vi "Mouse Down.vi"(8 "error in":errorcluster, 10 "Double Click":bool, 11 "Data in":T1={"Class"={"Ants"=refnum, "Layer"=refnum, "Templates"=refnum, "Icon"=refnum, "Glyph"=refnum, "Settings"=refnum, "Tools"=refnum}, "Ref"={"Add Layer"=refnum, "Remove Layer"=refnum, "Line Text"=[], "Body Text Spec"=refnum, "DNL_Font"=refnum, "glyph path str"=refnum, "templates path str"=refnum, "Arrow Up"=refnum, "Arrow Down"=refnum, "IE VI Ref"=refnum, "Glyphs tree"=refnum, "Templates tree"=refnum, "Layer Icon Text"=refnum, "Layer Template"=refnum, "Clipboard"=refnum, "BW icon in"=refnum, "Color icon in"=refnum, "Layer Clust"=refnum, "Body Text"=refnum, "DNL_Framework Templates"=refnum, "Search Templates"=refnum, "TextMarker"=refnum, "Tab Control"=refnum, "Search Glyphs"=refnum, "Line Color"=refnum, "DNL_Glyphs []"=refnum, "Fill Color"=refnum, "Tools"=refnum, "Glyphs tree"=refnum, "Icon"=refnum, "Preview"=refnum, "Ants"=refnum, "Terminals"=refnum, "menu reference"=refnum, "LayerNames"=[], "GlyphLoadAnimation"=refnum, "TemplateLoadAnimation"=refnum, "refreshGlyphs"=refnum, "refreshTemplates"=refnum}, "Support"={"AntsRect"={"left"=0, "top"=0, "right"=0, "bottom"=0}, "Mouse Move Coords"={"Horizontal"=0, "Vertical"=0}, "Mouse Down Coords"={"Horizontal"=0, "Vertical"=0}, "Temp Coord"={"Horizontal"=0, "Vertical"=0}, "Action"=enum."Default", "Edge Color"=4914962, "Fill Color"=16860, "Mouse Down?"=FALSE, "Draft Mode?"=FALSE, "Temp Icon"=bytes[3102], "CTRL Pressed"=FALSE, "Move Selection?"=FALSE, "AntsRect Orig"={"left"=0, "top"=0, "right"=0, "bottom"=0}, "Text"="", "TM Set?"=FALSE, "Mouse inside icon?"=FALSE, "Tool (old value)"=0, "Pencil Move Color"=0, "Swap Colors?"=FALSE, "Shift pressed?"=FALSE}}) -> (0 "error out":errorcluster, 3 "Data out":T1={"Class"={"Ants"=refnum, "Layer"=refnum, "Templates"=refnum, "Icon"=refnum, "Glyph"=refnum, "Settings"=refnum, "Tools"=refnum}, "Ref"={"Add Layer"=refnum, "Remove Layer"=refnum, "Line Text"=[], "Body Text Spec"=refnum, "DNL_Font"=refnum, "glyph path str"=refnum, "templates path str"=refnum, "Arrow Up"=refnum, "Arrow Down"=refnum, "IE VI Ref"=refnum, "Glyphs tree"=refnum, "Templates tree"=refnum, "Layer Icon Text"=refnum, "Layer Template"=refnum, "Clipboard"=refnum, "BW icon in"=refnum, "Color icon in"=refnum, "Layer Clust"=refnum, "Body Text"=refnum, "DNL_Framework Templates"=refnum, "Search Templates"=refnum, "TextMarker"=refnum, "Tab Control"=refnum, "Search Glyphs"=refnum, "Line Color"=refnum, "DNL_Glyphs []"=refnum, "Fill Color"=refnum, "Tools"=refnum, "Glyphs tree"=refnum, "Icon"=refnum, "Preview"=refnum, "Ants"=refnum, "Terminals"=refnum, "menu reference"=refnum, "LayerNames"=[], "GlyphLoadAnimation"=refnum, "TemplateLoadAnimation"=refnum, "refreshGlyphs"=refnum, "refreshTemplates"=refnum}, "Support"={"AntsRect"={"left"=0, "top"=0, "right"=0, "bottom"=0}, "Mouse Move Coords"={"Horizontal"=0, "Vertical"=0}, "Mouse Down Coords"={"Horizontal"=0, "Vertical"=0}, "Temp Coord"={"Horizontal"=0, "Vertical"=0}, "Action"=enum."Default", "Edge Color"=4914962, "Fill Color"=16860, "Mouse Down?"=FALSE, "Draft Mode?"=FALSE, "Temp Icon"=bytes[3102], "CTRL Pressed"=FALSE, "Move Selection?"=FALSE, "AntsRect Orig"={"left"=0, "top"=0, "right"=0, "bottom"=0}, "Text"="", "TM Set?"=FALSE, "Mouse inside icon?"=FALSE, "Tool (old value)"=0, "Pencil Move Color"=0, "Swap Colors?"=FALSE, "Shift pressed?"=FALSE}})   [LabVIEW 2021]
uses:
  <resource>/plugins/NIIconEditor/Controls/IE Data.ctl
  <resource>/plugins/NIIconEditor/Class/Ants/Ants.lvclass
  <resource>/plugins/NIIconEditor/Class/FakedArray/FakedArray.lvclass
  <resource>/plugins/NIIconEditor/Class/Icon Library/Glyph.lvclass
  <resource>/plugins/NIIconEditor/Class/Settings/Settings.lvclass
  <resource>/plugins/NIIconEditor/Class/Tools/Tools Paint.lvclass
  <vilib>/LabVIEW Icon API/lv_icon/Classes/Icon/Icon.lvclass
  <resource>/plugins/NIIconEditor/Controls/IE Classes.ctl
  <resource>/plugins/NIIconEditor/Controls/References Cluster.ctl
  <resource>/plugins/NIIconEditor/Controls/SupportClass.ctl
  <vilib>/Utility/miscctls.llb/LVPoint32TypeDef.ctl
  <resource>/plugins/NIIconEditor/Controls/SupportClass_Action.ctl
  <vilib>/LabVIEW Icon API/lv_icon/Controls/IEColor.ctl
  <vilib>/LabVIEW Icon API/lv_icon/Controls/LayerType.ctl
  <vilib>/LabVIEW Icon API/lv_icon/Classes/Layer/Layer.lvclass
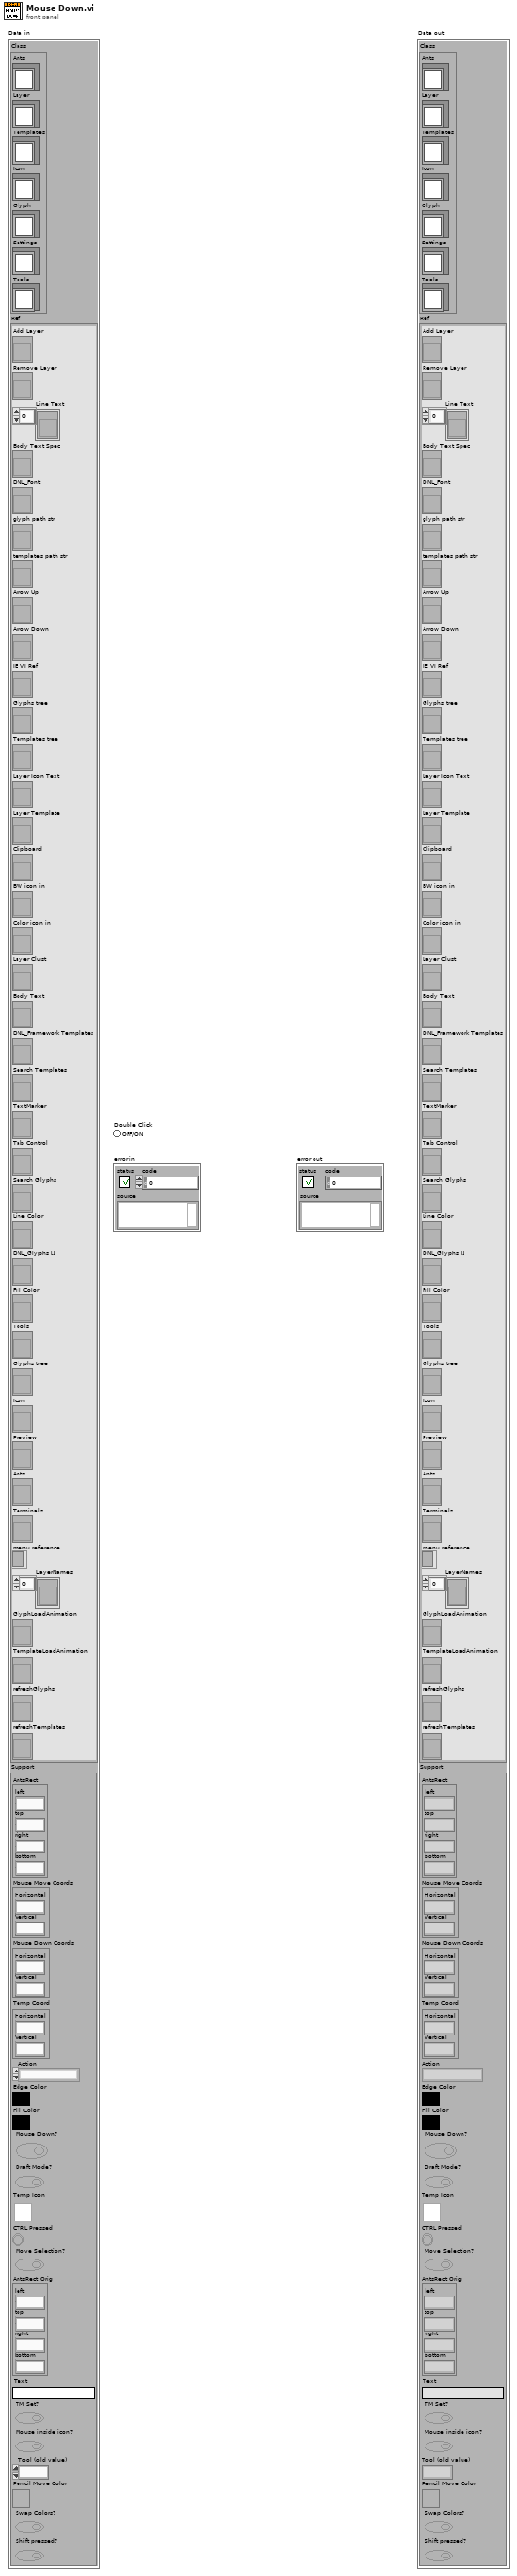
[diagram p1: front panel]
types:
  T1 = typedef "IE Data.ctl" = cluster{"Class":T2, "Ref":T3, "Support":T4}
  T2 = typedef "IE Classes.ctl" = cluster{"Ants":refnum<class "Ants.lvclass">, "Layer":refnum<class "FakedArray.lvclass">, "Templates":refnum<class "FakedArray.lvclass">, "Icon":refnum<class "Icon.lvclass">, "Glyph":refnum<class "Glyph.lvclass">, "Settings":refnum<class "Settings.lvclass">, "Tools":refnum<class "Tools Paint.lvclass">}
  T3 = typedef "References Cluster.ctl" = cluster{"Add Layer":refnum<vi>, "Remove Layer":refnum<vi>, "Line Text":refnum<vi>[], "Body Text Spec":refnum<vi>, "DNL_Font":refnum<vi>, "glyph path str":refnum<vi>, "templates path str":refnum<vi>, "Arrow Up":refnum<vi>, "Arrow Down":refnum<vi>, "IE VI Ref":refnum<vi>, "Glyphs tree":refnum<vi>, "Templates tree":refnum<vi>, "Layer Icon Text":refnum<vi>, "Layer Template":refnum<vi>, "Clipboard":refnum<vi>, "BW icon in":refnum<vi>, "Color icon in":refnum<vi>, "Layer Clust":refnum<vi>, "Body Text":refnum<vi>, "DNL_Framework Templates":refnum<vi>, "Search Templates":refnum<vi>, "TextMarker":refnum<vi>, "Tab Control":refnum<vi>, "Search Glyphs":refnum<vi>, "Line Color":refnum<vi>, "DNL_Glyphs []":refnum<vi>, "Fill Color":refnum<vi>, "Tools":refnum<vi>, "Glyphs tree":refnum<vi>, "Icon":refnum<vi>, "Preview":refnum<vi>, "Ants":refnum<vi>, "Terminals":refnum<vi>, "menu reference":refnum<k9>, "LayerNames":refnum<vi>[], "GlyphLoadAnimation":refnum<vi>, "TemplateLoadAnimation":refnum<vi>, "refreshGlyphs":refnum<vi>, "refreshTemplates":refnum<vi>}
  T4 = typedef "SupportClass.ctl" = cluster{"AntsRect":cluster{"left":i16, "top":i16, "right":i16, "bottom":i16}, "Mouse Move Coords":T5, "Mouse Down Coords":T5, "Temp Coord":T5, "Action":T6, "Edge Color":T7, "Fill Color":T7, "Mouse Down?":bool, "Draft Mode?":bool, "Temp Icon":picture, "CTRL Pressed":bool, "Move Selection?":bool, "AntsRect Orig":cluster{"left":i16, "top":i16, "right":i16, "bottom":i16}, "Text":string, "TM Set?":bool, "Mouse inside icon?":bool, "Tool (old value)":u32, "Pencil Move Color":u32, "Swap Colors?":bool, "Shift pressed?":bool}
  T5 = typedef "LVPoint32TypeDef.ctl" = cluster{"Horizontal":i32, "Vertical":i32}
  T6 = typedef "SupportClass_Action.ctl" = enum16{"Default", "Move Selection", "Glyph Library", "Tool"}
  T7 = typedef "IEColor.ctl" = u32
  T8 = typedef "LayerType.ctl" = enum16{"Graphic", "Text", "Tool", "Graphic Drop"}
  T9 = cluster{"left":i16, "top":i16, "right":i16, "bottom":i16}
  T10 = typedef "Tools.ctl" = enum32{"Pencil", "Line", "Dropper", "Fill", "Rectangle", "Filled Rectangle", "Ellipse", "Filled Ellipse", "Eraser", "Text", "Select", "Move"}
  T11 = typedef "INI.ctl" = cluster{"Show Layer Tab?":bool, "Show Terminals?":bool, "Text":cluster{"Font":T12, "Alignment":T13, "Size":T14}, "3rd party Templates":cluster{"Store 3rd party Templates?":bool, "Folder Name":string}, "Merge user layers on commit":bool, "Body Text":T15, "Fill Color":T7, "Edge Color":T7, "Tab":u16, "Tool":T10, "Disable Layers?":bool}
  T12 = typedef "Font.ctl" = string
  T13 = typedef "Alignment.ctl" = u16
  T14 = typedef "Font Size.ctl" = u8
  T15 = typedef "BodyText.ctl" = cluster{"Line 1 text":string, "Line 2 text":string, "Line 3 text":string, "Line 4 text":string, "Line 1 color":u32, "Line 2 color":u32, "Line 3 color":u32, "Line 4 color":u32, "Body Text Spec":cluster{"Font":T12, "Alignment":T13, "Size":u8}, "Center text vertically":bool, "Capitalize Text":bool}
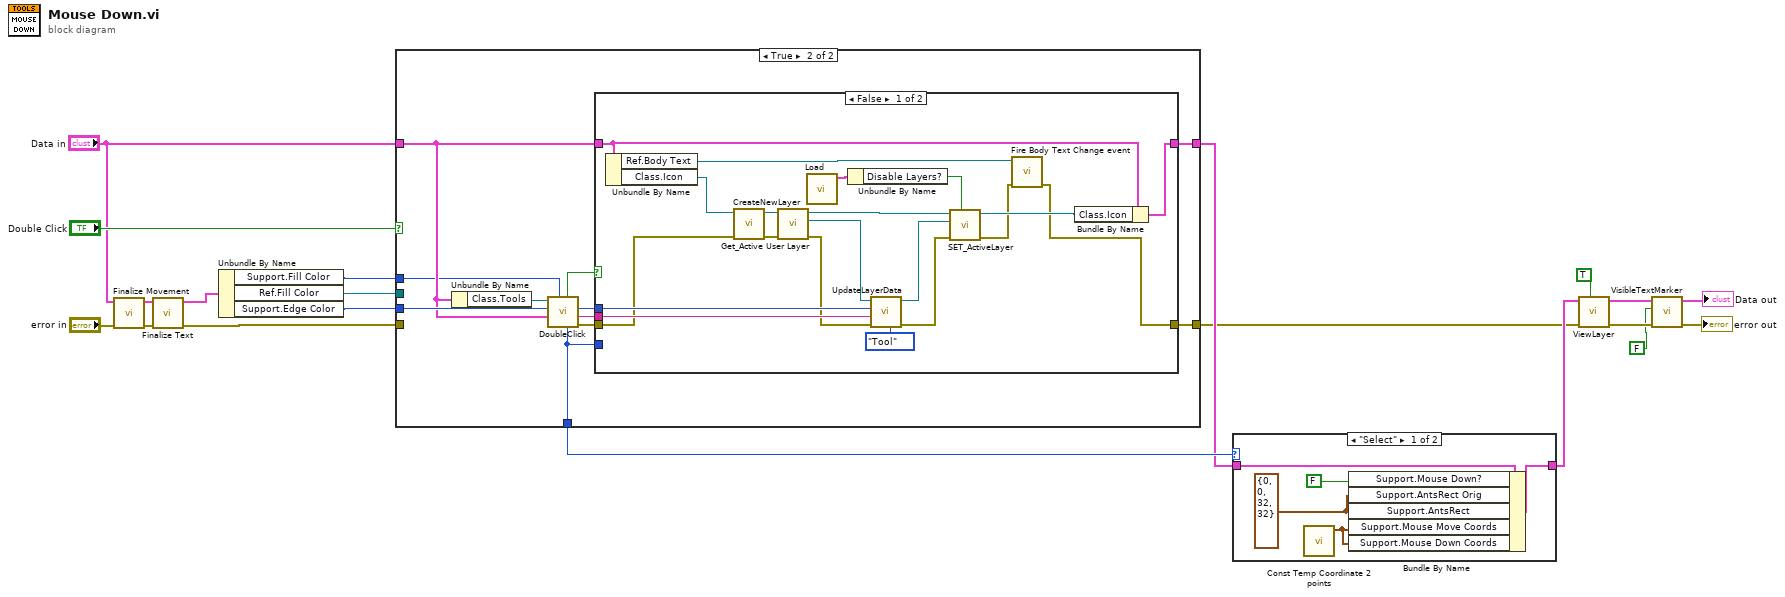
[diagram p0: block diagram]
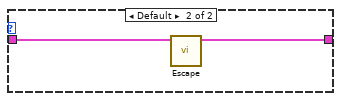
[diagram p2: hidden frame]
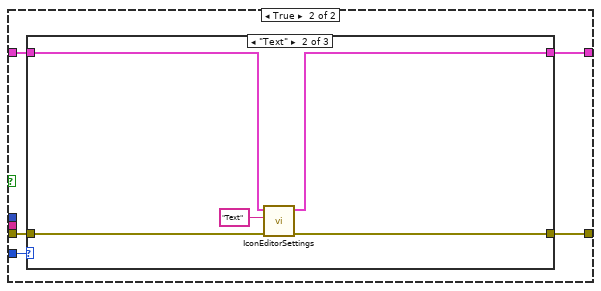
[diagram p4: hidden frame]
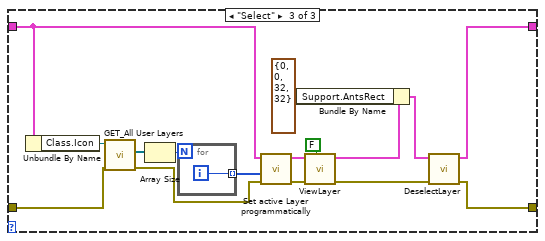
[diagram p6: hidden frame]
diagram:
  n1 = call <resource>:"Finalize Movement.vi"("error in (no error)"="error in", "Data in"="Data in") -> ("error out"=w13:errorcluster, "Data out"=w11:T1)  [unwired: 1 in, 7 out]
  n2 = call <resource>:"Finalize Text.vi"("error in (no error)"=w13, "Data in"=w11) -> ("error out"=w9:errorcluster, "Data out"=w10:T1)  [unwired: 8 out]
  n3 = Unbundle By Name(w10) -> ("Support.Fill Color"=w1:T7, "Ref.Fill Color"=w17:refnum<vi>, "Support.Edge Color"=w19:T7)
  n4 = case shown="True" "Double Click" {
    tunnel: w9 -> [w22 _]
    tunnel: w19 -> [_ w33]
    tunnel: [w22 w31] -> w2
    tunnel: [_ w27] -> w20
    tunnel: w17 -> [_ _]
    tunnel: "Data in" -> [w21 w25]
    tunnel: [w21 w24] -> w3
    tunnel: w1 -> [_ w23]
    frame False {
    }
    frame True {
      n5 = Unbundle By Name(w25) -> ("Class.Tools"=w26:refnum<class "Tools Paint.lvclass">)
      n6 = call <resource>:"DoubleClick.vi"("Fill Color"=w23, "Data in"=w25, "Edge Color"=w33, "Tools Paint in"=w26) -> ("error out"=w32:errorcluster, "Name"=w29:string, "new picture"=w30:picture, "Active Tool"=w27:T10, "Invalid Picture?"=w28:bool)  [unwired: 1 in, 2 out]
      n7 = case shown="False" w28 {
        tunnel: w32 -> [w50 w57]
        tunnel: [w37 w56] -> w31
        tunnel: w30 -> [w53 _]
        tunnel: w29 -> [w52 _]
        tunnel: w27 -> [_ w58]
        tunnel: w25 -> [w39 w55]
        tunnel: [w51 w54] -> w24
        frame False {
          n8 = Unbundle By Name(w39) -> ("Ref.Body Text"=w36:refnum<vi>, "Class.Icon"=w41:refnum<class "Icon.lvclass">)
          n9 = call <vilib>:"CreateNewLayer.vi"("error in"=w50, "Icon.lvclass"=w41) -> ("error out"=w49:errorcluster, "Icon.lvclass out"=w48:refnum<class "Icon.lvclass">)  [unwired: 3 in, 5 out]
          n10 = call-dynamic "Get_Active User Layer.vi"("error in (no error)"=w49, "Icon in"=w48) -> ("error out"=w46:errorcluster, "Layer.lvclass"=w45:refnum<class "Layer.lvclass">, "Icon out"=w47:refnum<class "Icon.lvclass">)  [unwired: 7 out]
          n11 = call <resource>:"Load.vi"() -> ("INI Data"=w35:T11)  [unwired: 2 in, 9 out]
          n12 = Unbundle By Name(w35) -> ("Disable Layers?"=w34:bool)
          n13 = call <vilib>:"UpdateLayerData.vi"("Type"=LayerType."Tool", "error in"=w46, "LayerName"=w52, "new picture"=w53, "Active Layer"=w45) -> ("error out"=w43:errorcluster, "Layer.lvclass out"=w44:refnum<class "Layer.lvclass">)  [unwired: 3 in, 2 out]
          n14 = call-dynamic "SET_ActiveLayer.vi"("Combine User Layers?"=w34, "error in (no error)"=w43, "Layer.lvclass"=w44, "Icon.lvclass in"=w47) -> ("error out"=w38:errorcluster, "Icon.lvclass out"=w40:refnum<class "Icon.lvclass">)  [unwired: 6 out]
          n15 = call <resource>:"Fire Body Text Change event.vi"("error in"=w38, "Ref.Body Text"=w36) -> ("error out"=w37:errorcluster)  [unwired: 2 in, 7 out]
          n16 = Bundle By Name(cluster=w39, "Class.Icon"=w40) -> (w51:T1)
        }
        frame True {
          n17 = case shown="\"Text\"" w58 {
            tunnel: w57 -> [w60 w65 w73]
            tunnel: [w60 w62 w66] -> w56
            tunnel: w55 -> [w59 w63 w72]
            tunnel: [w59 w61 w67] -> w54
            frame "Ellipse", Default {
            }
            frame "Text" {
              n18 = call <resource>:"IconEditorSettings.vi"("error in (no error)"=w65, "Active Tag"="Text", "Data in"=w63) -> ("error out"=w62:errorcluster, "Data out"=w61:T1)  [unwired: 7 out]
            }
            frame "Select" {
              n19 = Unbundle By Name(w72) -> ("Class.Icon"=w71:refnum<class "Icon.lvclass">)
              n20 = call-dynamic "GET_All User Layers.vi"("error in (no error)"=w73, "Icon.lvclass in"=w71) -> ("error out"=w78:errorcluster, "User Layer"=w81:refnum<class "Layer.lvclass">[])  [unwired: 7 in, 1 out]
              n21 = Array Size(array=w81) -> (size(s)=w80:i32)
              n22 = for {
                N: w80 -> [_]
                tunnel: [w82] -> w79 mode=indexing
                i -> [w82]
              }
              n23 = call <resource>:"Set active Layer programmatically.vi"("error in"=w78, "Active Layer []"=w79, "Data in"=w72) -> ("error out"=w75:errorcluster, "Data out"=w76:T1)  [unwired: 7 in]
              n24 = call <resource>:"ViewLayer.vi"("Add to Undo?"=FALSE, "error in (no error)"=w75, "Data in"=w76) -> ("error out"=w68:errorcluster, "Data out"=w70:T1)  [unwired: 1 in, 6 out]
              n25 = Bundle By Name(cluster=w70, "Support.AntsRect"=T9 {"left"=0, "top"=0, "right"=32, "bottom"=32}) -> (w69:T1)
              n26 = call <resource>:"DeselectLayer.vi"("error in (no error)"=w68, "Data in"=w69) -> ("error out"=w66:errorcluster, "Data out"=w67:T1)  [unwired: 8 out]
            }
          }
        }
      }
    }
  }
  n27 = case shown="\"Select\"" w20 {
    tunnel: w3 -> [w85 w89]
    tunnel: [w84 w88] -> w7
    frame "Select" {
      w83 = T9 {"left"=0, "top"=0, "right"=32, "bottom"=32} ("Support.AntsRect Orig")
      n28 = call <resource>:"Const Temp Coordinate 2 points.vi"() -> ("Const Temp Coordinate"=w86:T5)  [unwired: 11 out]
      n29 = Bundle By Name(cluster=w85, "Support.Mouse Down?"=FALSE ("Mouse Down?"), "Support.AntsRect Orig"=w83, "Support.AntsRect"=w83, "Support.Mouse Move Coords"=w86, "Support.Mouse Down Coords"=w86) -> (w84:T1)
    }
    frame Default {
      n30 = call <resource>:"Escape.vi"("Data in"=w89) -> ("Data out"=w88:T1)  [unwired: 2 in, 8 out]
    }
  }
  n31 = call <resource>:"ViewLayer.vi"("Add to Undo?"=TRUE, "error in (no error)"=w2, "Data in"=w7) -> ("error out"=w15:errorcluster, "Data out"=w6:T1)  [unwired: 2 in, 5 out]
  n32 = call <resource>:"VisibleTextMarker.vi"("error in (no error)"=w15, "Visible"=FALSE, "Data in"=w6) -> ("error out"=→"error out":errorcluster, "Data out"=→"Data out":T1)  [unwired: 1 in, 6 out]
